vi "Get_Subset.vi"(8 "index":i32=5000, 11 "Input":dbl[][](array[numeric])) -> (3 "Output":dbl[][](array[numeric]))   [LabVIEW 2020]
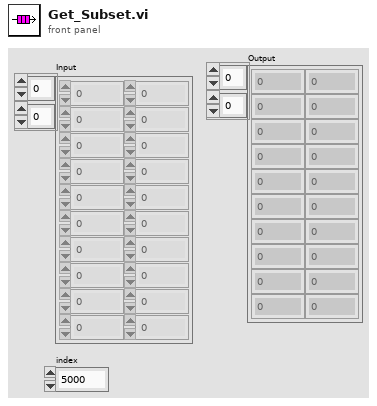
[diagram p1: front panel]
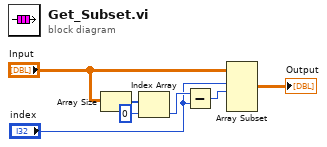
[diagram p0: block diagram]
diagram:
  n1 = Array Size(array="Input") -> (size(s)=w7:i32[])
  n2 = Index Array(array=w7, index=0) -> (element=w5:i32)
  n3 = Subtract(x=w5, y="index") -> (x-y=w1:i32)
  n4 = Array Subset(array="Input", index (row)="index", length (row)=w1) -> (→"Output":dbl[][])  [unwired: 2 in]
